vi "Build from ProjFile GObject Entry.vi"(8 "error in (no error)":errorcluster, 10 "ProjFile Entry":T1, 11 "GObject in":refnum<class "GObject.lvclass">) -> (0 "error out":errorcluster, 3 "GObject out":refnum<class "GObject.lvclass">)   [LabVIEW 2013, in "SET Project Data.lvlib" / "GObject.lvclass"]
uses:
  GObject.lvclass
  Types/ProjFile_GObject Data.ctl
  GObject.lvclass/GObject.ctl
  SET Project Data.lvlib
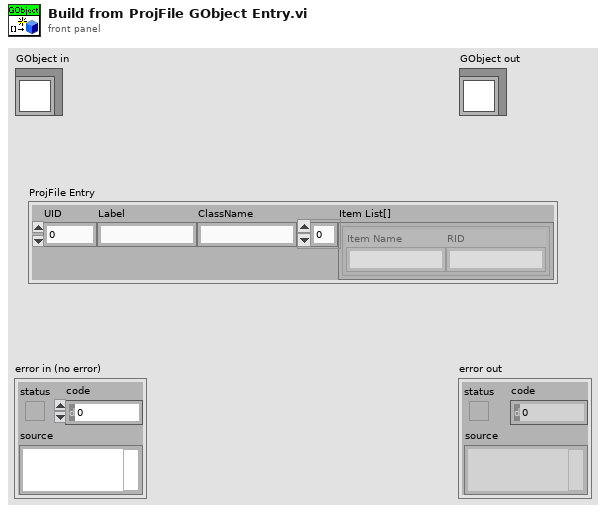
[diagram p1: front panel]
types:
  T1 = typedef "SET Project Data.lvlib/ProjFile_GObject Data.ctl" = cluster{"UID":i32, "Label":string, "ClassName":string, "Item List[]":cluster{"Item Name":string, "RID":string}[]}
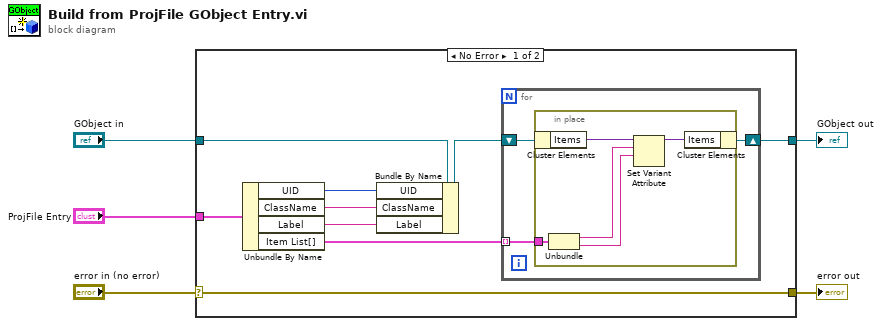
[diagram p0: block diagram]
diagram:
  n1 = case shown="No Error" "error in (no error)" {
    selector: "error in (no error)" -> [w14 w24]
    tunnel: [w14 w24] -> w4
    tunnel: [w11 w23] -> w2
    tunnel: "GObject in" -> [w13 w23]
    tunnel: "ProjFile Entry" -> [w10 _]
    frame No Error {
      n2 = Unbundle By Name(w10) -> ("UID"=w9:i32, "ClassName"=w8:string, "Label"=w7:string, "Item List[]"=w6:cluster{"Item Name":string, "RID":string}[])
      n3 = Bundle By Name(cluster=w13, "UID"=w9, "ClassName"=w8, "Label"=w7) -> (w12:refnum<class "GObject.lvclass">)
      n4 = for {
        shift-right: [w16] -> w11
        shift-left: w12 -> [w17]
        tunnel: w6 -> [w15] mode=indexing
        n5 = in-place {
          in-place-border: w15 -> [w20]
          n6 = in-place-cluster #1(w17) -> ("Items"=w22:variant)
          n7 = Unbundle(w20) -> ("Item Name"=w19:string, "RID"=w18:string)
          n8 = Set Variant Attribute(Variant=w22, name=w19, value=w18) -> (Variant out=w21:variant)  [unwired: 1 in, 2 out]
          n9 = in-place-cluster #1("Items"=w21) -> (w16:refnum<class "GObject.lvclass">)
        }
      }
    }
    frame Error {
    }
  }
  "error out" <- w4
  "GObject out" <- w2
